vi "Begin.vi"(8 "error in":errorcluster) -> (0 "error out":errorcluster)   [LabVIEW 2017]
doc: "Called before other user functions, this VI is expected to open initial I/O refnums, load in file data, and do all program initialization. Notice that the <B>error out</B> terminal is simply used for data flow. Wiring it to other structures or subVIs ensures that this VI runs first."
uses:
  <vilib>/Rock Robotics/WPI/MotorControl/WPI_MotorControlDeviceRef.ctl
  <vilib>/Rock Robotics/WPI/MotorControl/WPI_MotorControlType.ctl
  <vilib>/Rock Robotics/SystemInterfaces/DIO/FPGA_DIOPWMChannel.ctl
  <vilib>/Rock Robotics/WPI/PWM/WPI_PWMDeadband.ctl
  <vilib>/Rock Robotics/SystemInterfaces/DIO/FPGA_DIOChannel.ctl
  <vilib>/Rock Robotics/WPI/DriverStation/WPI_DriverStationRobotMode2.ctl
  SwerveLibrary/Swerve Motors.ctl
  SwerveLibrary/Drive Motors.ctl
  SwerveLibrary/Controllers.ctl
  <vilib>/Rock Robotics/WPI/Joystick/WPI_JoystickDeviceEnum.ctl
  Arm Control/Arm Motor.ctl
  <vilib>/Rock Robotics/WPI/Solenoid/WPI_SolenoidChannel.ctl
  <vilib>/Rock Robotics/WPI/SafetyOutput/WPI_SafetyOutputConfigMenu.ctl
  Public/Documents/Cross The Road Electronics/Phoenix-LabVIEW/Motor Controller/Controls/CTRE_Phoenix_MotorControl_FeedbackDevice.ctl
  Pigeon IMU.ctl
  Robot Global Data.vi
  <vilib>/Rock Robotics/WPI/ThirdParty/Phoenix-LabVIEW/Pigeon IMU/CTRE_PigeonIMU_Open_CAN.vi
  Public/Documents/Cross The Road Electronics/Phoenix-LabVIEW/Pigeon IMU/CTRE_PigeonIMU_GetYPR.vi
  <vilib>/Rock Robotics/WPI/ThirdParty/Phoenix-LabVIEW/Motor Controller/Get/CTRE_Phoenix_MotorController_GetPulseWidthAll.vi
  <vilib>/Rock Robotics/WPI/Utilities/WPI_GetSetVariantRefNum.vi
  <vilib>/Rock Robotics/WPI/Solenoid/WPI_SolenoidOpenSingle.vi
  SwerveLibrary/Huskie Swerve.lvlib
panel:
  out "PhoenixMotorControlDevRef":T1={"DeviceStatus"={"status"=FALSE, "code"=0, "source"=""}, "Type"=enum."PWM", "PWM"={"PWM Channel"=enum."Invalid", "DeadBand"={"Name"="", "maxPositivePwm"=0, "minPositivePwm"=0, "centerPwm"=0, "maxNegativePwm"=0, "minNegativePwm"=0, "angularRange"=0}}, "CAN"={"Device Number"=0, "SetOutput VI Ref"=variant(refnum<vi> refnum), "GetOutput VI Ref"=variant(refnum<vi> refnum), "Enable VI Ref"=variant(refnum<vi> refnum), "Disable VI Ref"=variant(refnum<vi> refnum), "Data"=variant}, "Invert"=FALSE, "DIO PWM"={"PWM \"Enable\" Channel"=enum."Invalid", "DIOChannel"=enum."Invalid", "PWM Rate"=0.0}}
  out "Yaw Pitch Roll":cluster{"Yaw":dbl, "Pitch":dbl, "Roll":dbl}
  in  "PID gains":T6={"proportional gain (Kc)"=5.0, "integral time (Ti, min)"=0.0, "derivative time (Td, min)"=0.0} {"derivative time (Td, min)" format="%.3f"; "integral time (Ti, min)" format="%.8f"; "proportional gain (Kc)" format="%.8f"}
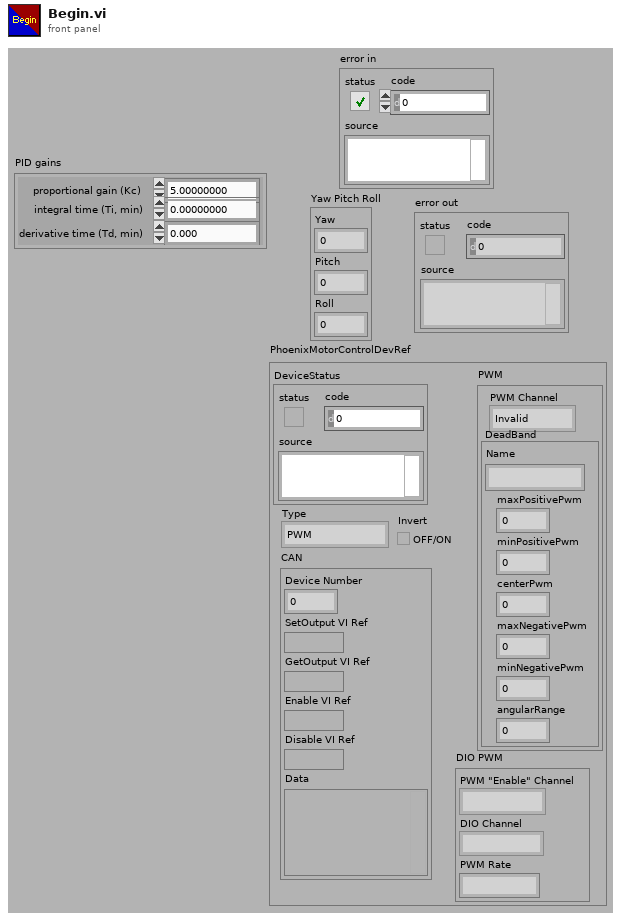
[diagram p1: front panel]
types:
  T1 = typedef "WPI_MotorControlDeviceRef.ctl" = cluster{"DeviceStatus":errorcluster, "Type":T2, "PWM":cluster{"PWM Channel":T3, "DeadBand":T4}, "CAN":cluster{"Device Number":u8, "SetOutput VI Ref":variant, "GetOutput VI Ref":variant, "Enable VI Ref":variant, "Disable VI Ref":variant, "Data":variant}, "Invert":bool, "DIO PWM":cluster{"PWM \"Enable\" Channel":T3, "DIOChannel":T5, "PWM Rate":dbl}}
  T2 = typedef "WPI_MotorControlType.ctl" = enum16{"PWM", "CAN", "DIO PWM"}
  T3 = typedef "FPGA_DIOPWMChannel.ctl" = enum8{"PWM 0", "PWM 1", "PWM 2", "PWM 3", "PWM 4", "PWM 5", "PWM 6", "PWM 7", "PWM 8", "PWM 9", "PWM MXP 0", "PWM MXP 1", "PWM MXP 2", "PWM MXP 3", "PWM MXP 4", "PWM MXP 5", "PWM MXP 6", "PWM MXP 7", "PWM MXP 8", "PWM MXP 9", "Invalid"}
  T4 = typedef "WPI_PWMDeadband.ctl" = cluster{"Name":string, "maxPositivePwm":i32, "minPositivePwm":i32, "centerPwm":i32, "maxNegativePwm":i32, "minNegativePwm":i32, "angularRange":u16}
  T5 = typedef "FPGA_DIOChannel.ctl" = enum8{"DIO 0", "DIO 1", "DIO 2", "DIO 3", "DIO 4", "DIO 5", "DIO 6", "DIO 7", "DIO 8", "DIO 9", "DIO MXP 0", "DIO MXP 1", "DIO MXP 2", "DIO MXP 3", "DIO MXP 4", "DIO MXP 5", "DIO MXP 6", "DIO MXP 7", "DIO MXP 8", "DIO MXP 9", "DIO MXP 10", "DIO MXP 11", "DIO MXP 12", "DIO MXP 13", "DIO MXP 14", "DIO MXP 15", "SPI Port CS1", "SPI Port CS2", "SPI Port CS3", "SPI Port MISO", "SPI Port MOSI", "Invalid"}
  T6 = cluster{"proportional gain (Kc)":dbl, "integral time (Ti, min)":dbl, "derivative time (Td, min)":dbl}
  T7 = typedef "WPI_SolenoidChannel.ctl" = enum8{"Solenoid 0", "Solenoid 1", "Solenoid 2", "Solenoid 3", "Solenoid 4", "Solenoid 5", "Solenoid 6", "Solenoid 7", "Invalid"}
  T8 = enum16{"Shoulder", "Forearm", "Grabber", "Extra"}[]
  T9 = typedef "Arm Motor.ctl" = enum16{"Shoulder Motor", "Forearm Motor"}
  T10 = typedef "WPI_JoystickDeviceEnum.ctl" = enum16{"USB 0", "USB 1", "USB 2", "USB 3", "USB 4", "USB 5"}
  T11 = typedef "Huskie Swerve.lvlib/Controllers.ctl" = enum16{"Joystick", "Buttons"}
  T12 = typedef "Huskie Swerve.lvlib/Drive Motors.ctl" = enum16{"Drive 1", "Drive 2", "Drive 3", "Drive 4"}
  T13 = typedef "Huskie Swerve.lvlib/Swerve Motors.ctl" = enum16{"Swerve 1", "Swerve 2", "Swerve 3", "Swerve 4"}
  T14 = typedef "WPI_DriverStationRobotMode2.ctl" = enum16{"Autonomous Disabled", "Autonomous Enabled", "Teleop Disabled", "Teleop Enabled", "Disconnected", "Finish", "Test Disabled", "Test Enabled", "Emergency Stopped"}
  T15 = typedef "WPI_SafetyOutputConfigMenu.ctl" = enum16{"Enable", "Disable"}
  T16 = typedef "CTRE_Phoenix_MotorControl_FeedbackDevice.ctl" = i8
  T17 = typedef "WPI_JoystickDevRef.ctl" = cluster{"Device":T10}
  T18 = typedef "Pigeon IMU.ctl" = enum16{"Pigeon IMU"}
  T19 = typedef "CTRE_PigeonIMU_DeviceRef.ctl" = cluster{"DeviceStatus":errorcluster, "Device Number":u8, "Type":T20, "Device ID":u32, "Handle":u64, "UsageFrame":u32, "Library Path":path}
  T20 = typedef "CTRE_PigeonIMU_ConnectionType.ctl" = u32
  T21 = typedef "WPI_CompressorDevRef.ctl" = cluster{"DevStatus":errorcluster, "Pneumatics Control Module":u8}
  T22 = typedef "WPI_SolenoidDevRef.ctl" = cluster{"DevStatus":errorcluster, "Pneumatics Control Module":u8, "Forward Solenoid Channel":T7, "Reverse Solenoid Channel":T7}
  T23 = typedef "WPI_DigitalInputDevRef.ctl" = cluster{"DevStatus":errorcluster, "DIO Channel":T5}
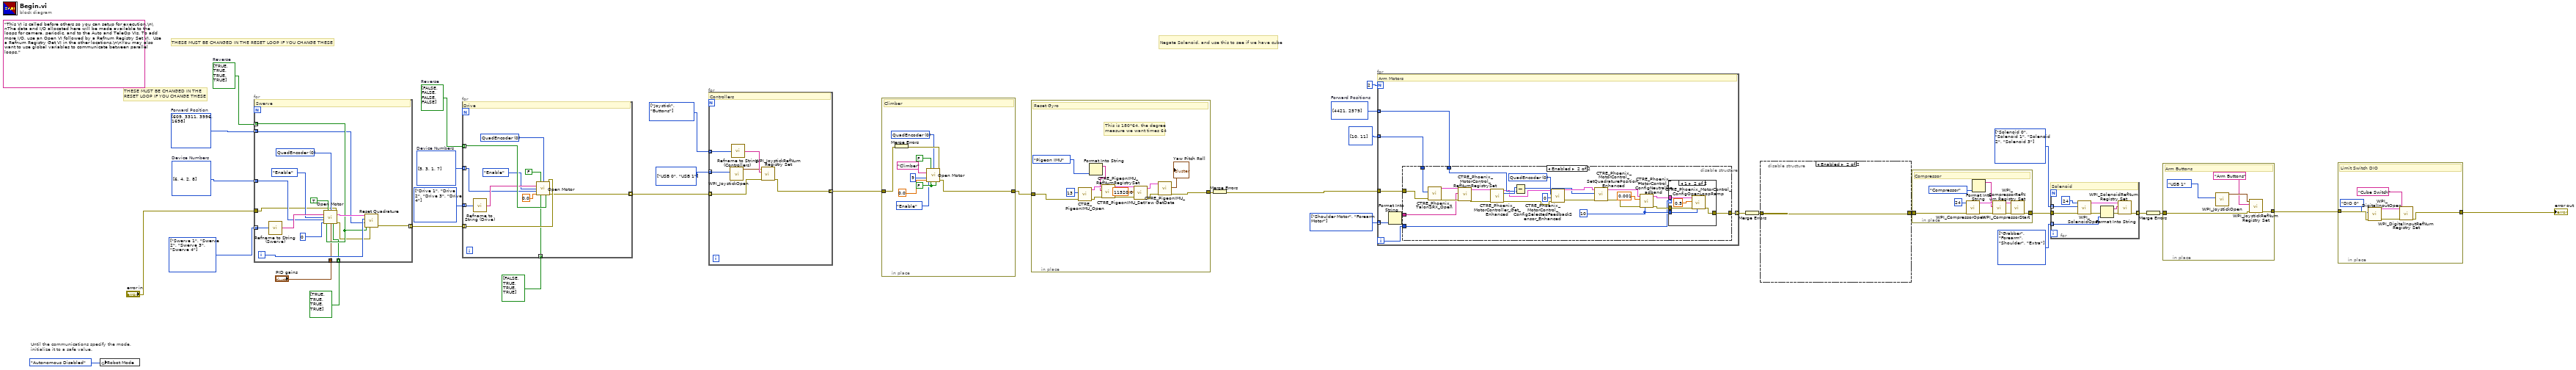
[diagram p0: block diagram]
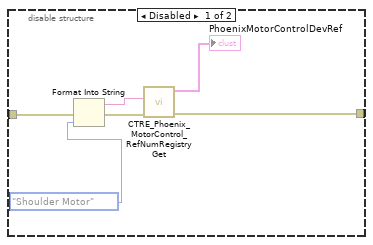
[diagram p2: hidden frame]
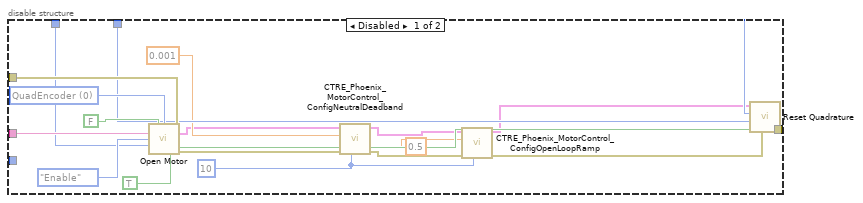
[diagram p3: hidden frame]
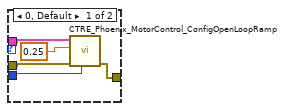
[diagram p4: hidden frame]
diagram:
  w8 = T7[] [enum."Solenoid 0", enum."Solenoid 1", enum."Solenoid 2", enum."Solenoid 3"] items=["Solenoid 0", "Solenoid 1", "Solenoid 2", "Solenoid 3", "Solenoid 4", "Solenoid 5", "Solenoid 6", "Solenoid 7", "Invalid"]
  w9 = T8 [enum."Grabber", enum."Forearm", enum."Shoulder", enum."Extra"] items=["Shoulder", "Forearm", "Grabber", "Extra"]
  w12 = T9[] [enum."Shoulder Motor", enum."Forearm Motor"] items=["Shoulder Motor", "Forearm Motor"]
  w15 = i32[] [4421, 2579]  # Forward Positions
  w22 = T10[] [enum."USB 0", enum."USB 1"] items=["USB 0", "USB 1", "USB 2", "USB 3", "USB 4", "USB 5"]
  w23 = T11[] [enum."Joystick", enum."Buttons"] items=["Joystick", "Buttons"]
  w25 = T12[] [enum."Drive 1", enum."Drive 2", enum."Drive 3", enum."Drive 4"] items=["Drive 1", "Drive 2", "Drive 3", "Drive 4"]
  w27 = i32[] [5, 3, 1, 7]  # Device Numbers
  w28 = bool[] [FALSE, FALSE, FALSE, FALSE]  # Reverse
  w29 = bool[] [TRUE, TRUE, TRUE, TRUE]  # Reverse
  w30 = T13[] [enum."Swerve 1", enum."Swerve 2", enum."Swerve 3", enum."Swerve 4"] items=["Swerve 1", "Swerve 2", "Swerve 3", "Swerve 4"]
  w31 = i32[] [6, 4, 2, 8]  # Device Numbers
  w33 = i32[] [609, 3311, 3996, 1698]  # Forward Position
  (unwired) "This VI is called before others so you can setup for execution.\n\nThe data and I/O allocated here will be made available to the loops for camera, periodic, and to the Auto and TeleOp VIs. To add more I/O, use an Open VI followed by a Refnum Registry Set VI.  Use a Refnum Registry Get VI in the other locations.\n\nYou may also want to use global variables to communicate between parallel loops."
  # "THESE MUST BE CHANGED IN THE \nRESET LOOP IF YOU CHANGE THESE"
  # "THESE MUST BE CHANGED IN THE RESET LOOP IF YOU CHANGE THESE"
  # "Negate Solenoid, and use this to see if we have cube"
  # "Until the communications specify the mode,\ninitialize it to a safe value."
  n1 = global write "Robot Global Data.vi" "Robot Mode"(WPI_DriverStationRobotMode2."Autonomous Disabled" ("Robot Mode")) -> ()
  n2 = for {
    tunnel: w33 -> [w39] mode=indexing
    tunnel: "error in" -> [w43]
    tunnel: w31 -> [w48] mode=indexing
    tunnel: w30 -> [w50] mode=indexing
    tunnel: w29 -> [w40] mode=indexing
    tunnel: [w37] -> w26 mode=indexing
    tunnel: "PID gains" -> [w36]
    tunnel: bool[] [TRUE, TRUE, TRUE, TRUE] -> [w35] mode=indexing
    i -> [w41]
    w44 = T16 0 items=["None"=-1, "QuadEncoder"=0, "Analog"=2, "Tachometer"=4, "Pulse Width Encoded Position"=8, "Sensor Sum (S0 + S1)"=9, "Sensor Difference (D0 - D1)"=10, "Remote Source 0"=11, "Remote Source 1"=12, "Software Emulated"=15] ("Feedback Reference")
    # "Swerve"
    n3 = call "Refname to String (Swerve).vi"("Enum"=w50) -> ("String"=w49:string)
    n4 = call "Open Motor.vi"("PID?"=TRUE, "Feedback Reference"=w44, "error in"=w43, "refnum name"=w49, "mode (safety config)"=WPI_SafetyOutputConfigMenu."Enable", "CAN Device Number"=w48, "Set sensor position"=0, "Reverse Feedback Sensor"=w40, "PID gains"=w36, "Invert Power"=w35) -> ("CAN Talon SRX Ref"=w42:T1, "error out"=w38:errorcluster)  [unwired: 4 in]
    n5 = call "Reset Quadrature.vi"("error in"=w38, "Reverse?"=w40, "Forward Position"=w39, "Module Number"=w41, "CAN Talon SRX Ref"=w42) -> ("error out"=w37:errorcluster)  [unwired: 5 in, 1 out]
  }
  n6 = for {
    tunnel: [w52] -> w24 mode=indexing
    tunnel: w28 -> [w60] mode=indexing
    tunnel: w27 -> [w58] mode=indexing
    tunnel: w26 -> [w53] mode=indexing
    tunnel: w25 -> [w61] mode=indexing
    tunnel: bool[] [FALSE, TRUE, TRUE, TRUE] ("Reverse Feedback Sensor") -> [w51] mode=indexing
    w54 = T16 0 items=["None"=-1, "QuadEncoder"=0, "Analog"=2, "Tachometer"=4, "Pulse Width Encoded Position"=8, "Sensor Sum (S0 + S1)"=9, "Sensor Difference (D0 - D1)"=10, "Remote Source 0"=11, "Remote Source 1"=12, "Software Emulated"=15] ("Feedback Reference")
    # "Drive"
    n7 = call "Refname to String (Drive).vi"("Enum"=w61) -> ("resulting string"=w59:string)
    n8 = call "Open Motor.vi"("PID?"=FALSE, "Feedback Reference"=w54, "error in"=w53, "refnum name"=w59, "mode (safety config)"=WPI_SafetyOutputConfigMenu."Enable", "CAN Device Number"=w58, "Set sensor position"=0.0, "Reverse Feedback Sensor"=w51, "Invert Power"=w60) -> ("error out"=w52:errorcluster)  [unwired: 5 in, 1 out]
  }
  n9 = for {
    tunnel: [w62] -> w18 mode=indexing
    tunnel: w24 -> [w63] mode=indexing
    tunnel: w23 -> [w66] mode=indexing
    tunnel: w22 -> [w67] mode=indexing
    # "Controllers"
    n10 = call <vilib>:"WPI_JoystickOpen.vi"("JoystickDevice"=w67) -> ("JoystickDevRef"=w64:T17)  [unwired: 10 in]
    n11 = call "Refname to String (Controllers).vi"("Enum"=w66) -> ("resulting string"=w65:string)
    n12 = call <vilib>:"WPI_JoystickRefNum Registry Set.vi"("error in (no error)"=w63, "refnum name"=w65, "JoystickDevRef"=w64) -> ("error out"=w62:errorcluster)  [unwired: 7 in, 1 out]
  }
  n13 = in-place "In Place Element Structure" {
    in-place-border: w18 -> [w76]
    in-place-border: [w68] -> w17
    w72 = T16 0 items=["None"=-1, "QuadEncoder"=0, "Analog"=2, "Tachometer"=4, "Pulse Width Encoded Position"=8, "Sensor Sum (S0 + S1)"=9, "Sensor Difference (D0 - D1)"=10, "Remote Source 0"=11, "Remote Source 1"=12, "Software Emulated"=15] ("Feedback Reference")
    w73 = FALSE ("Reverse Feedback Sensor")
    # "Climber"
    n14 = Merge Errors(w76) -> (w75:errorcluster)
    n15 = call "Open Motor.vi"("PID?"=FALSE, "Feedback Reference"=w72, "error in"=w75, "refnum name"="Climber", "mode (safety config)"=WPI_SafetyOutputConfigMenu."Enable", "CAN Device Number"=u8 9, "Set sensor position"=0.0, "Reverse Feedback Sensor"=w73, "Invert Power"=w73) -> ("error out"=w68:errorcluster)  [unwired: 5 in, 1 out]
  }
  n16 = in-place {
    in-place-border: w17 -> [w89]
    in-place-border: [w79] -> w16
    # "This is 180*64, the degree\nmeasure we want times 64"
    # "Reset Gyro"
    n17 = call-poly <vilib>:"CTRE_PigeonIMU_Open.vi"("error in"=w89, "Device Number"=u8 13) -> ("error out"=w87:errorcluster, "PigeonIMUDevRef"=w86:T19)  [unwired: 8 in]
    n18 = Format Into String(Pigeon_IMU."Pigeon IMU") -> (resulting string=w85:string)  [unwired: 3 in, 1 out]
    n19 = call <vilib>:"CTRE_PigeonIMU_RefNumRegistrySet.vi"("error in (no error)"=w87, "refnum name"=w85, "PigeonIMUDevRef"=w86) -> ("error out"=w84:errorcluster, "PigeonIMUDevRef"=w83:T19)  [unwired: 7 in]
    n20 = call <vilib>:"CTRE_PigeonIMU_SetYaw.vi"("error in (no error)"=w84, "Value"=11520.0, "PigeonIMUDevRef"=w83) -> ("error out"=w80:errorcluster, "PigeonIMUDevRef"=w81:T19)  [unwired: 7 in]
    n21 = call-poly "CTRE_PigeonIMU_GetData.vi"("error in (no error)"=w80, "PigeonIMUDevRef"=w81) -> ("error out"=w79:errorcluster, "Yaw Pitch Roll"=→"Yaw Pitch Roll":cluster{"Yaw":dbl, "Pitch":dbl, "Roll":dbl})  [unwired: 7 in, 1 out]
  }
  n22 = Merge Errors(w16) -> (w3:errorcluster)
  n23 = for {
    N: 2 -> [_]
    tunnel: w3 -> [w97]
    tunnel: w15 -> [w94] mode=indexing
    tunnel: i32[] [10, 11] -> [w93] mode=indexing
    tunnel: w12 -> [w95] mode=indexing
    tunnel: [w92] -> w7 mode=indexing
    i -> [w91]
    # "Arm Motors"
    n24 = Format Into String(w95) -> (resulting string=w96:string)  [unwired: 3 in, 1 out]
    n25 = disable-structure shown="Enabled" {
      disable-tunnel: w97 -> [w116 w139]
      disable-tunnel: w96 -> [w113 w136]
      disable-tunnel: w94 -> [w109 w130]
      disable-tunnel: w93 -> [w108 w140]
      disable-tunnel: [w104 w119] -> w92
      disable-tunnel: w91 -> [_ w117]
      frame Disabled {
        w100 = u32 10 ("timeoutMs")
        w114 = T16 0 items=["None"=-1, "QuadEncoder"=0, "Analog"=2, "Tachometer"=4, "Pulse Width Encoded Position"=8, "Sensor Sum (S0 + S1)"=9, "Sensor Difference (D0 - D1)"=10, "Remote Source 0"=11, "Remote Source 1"=12, "Software Emulated"=15] ("Feedback Reference")
        n26 = call "Open Motor.vi"("PID?"=FALSE, "Feedback Reference"=w114, "error in"=w116, "refnum name"=w113, "mode (safety config)"=WPI_SafetyOutputConfigMenu."Enable", "CAN Device Number"=w108, "Invert Power"=TRUE) -> ("CAN Talon SRX Ref"=w106:T1, "Reverse Feedback Sensor"=w110:bool, "error out"=w105:errorcluster)  [unwired: 6 in]
        n27 = call <vilib>:"CTRE_Phoenix_MotorControl_ConfigNeutralDeadband.vi"("timeoutMs"=w100, "error in (no error)"=w105, "Percent Deadband"=0.001, "PhoenixMotorControlDevRef"=w106) -> ("error out"=w103:errorcluster, "PhoenixMotorControlDevRef"=w101:T1)  [unwired: 6 in]
        n28 = call <vilib>:"CTRE_Phoenix_MotorControl_ConfigOpenLoopRamp.vi"("timeoutMs"=w100, "error in (no error)"=w103, "secondsFromNeutralToFull"=0.5, "PhoenixMotorControlDevRef"=w101) -> ("error out"=w102:errorcluster, "PhoenixMotorControlDevRef"=w98:T1)  [unwired: 6 in]
        n29 = call "Reset Quadrature.vi"("error in"=w102, "Reverse?"=w110, "Forward Position"=w109, "Module Number"=w108, "CAN Talon SRX Ref"=w98) -> ("error out"=w104:errorcluster)  [unwired: 5 in, 1 out]
      }
      frame Enabled {
        w123 = u32 10 ("timeoutMs")
        w135 = T16 0 items=["None"=-1, "QuadEncoder"=0, "Analog"=2, "Tachometer"=4, "Pulse Width Encoded Position"=8, "Sensor Sum (S0 + S1)"=9, "Sensor Difference (D0 - D1)"=10, "Remote Source 0"=11, "Remote Source 1"=12, "Software Emulated"=15] ("Feedback Device")
        n30 = call "CTRE_Phoenix_TalonSRX_Open.vi"("error in"=w139, "Device Number"=w140) -> ("error out"=w138:errorcluster, "CAN Talon SRX Ref"=w137:T1)  [unwired: 8 in]
        n31 = call <vilib>:"CTRE_Phoenix_MotorControl_RefNumRegistrySet.vi"("error in (no error)"=w138, "refnum name"=w136, "PhoenixMotorControlDevRef"=w137) -> ("error out"=w126:errorcluster, "PhoenixMotorControlDevRef"=w125:T1)  [unwired: 7 in]
        n32 = call-poly <vilib>:"CTRE_Phoenix_MotorController_Get_Enhanced.vi"("PhoenixMotorControlDevRef"=w125, "error in"=w126) -> ("PhoenixMotorControlDevRef"=w129:T1, "Pulse Width Position"=w131:i32, "error out"=w127:errorcluster)  [unwired: 8 in, 3 out]
        n33 = Subtract(x=w131, y=w130) -> (x-y=w128:i32)
        n34 = call "CTRE_Phoenix_MotorControl_ConfigSelectedFeedbackSensor_Enhanced.vi"("error in (no error)"=w127, "pidLoopIdx"=0, "Feedback Device"=w135, "PhoenixMotorControlDevRef"=w129) -> ("error out"=w132:errorcluster, "PhoenixMotorControlDevRef"=w133:T1)  [unwired: 6 in]
        n35 = call <vilib>:"CTRE_Phoenix_MotorControl_SetQuadraturePosition_Enhanced.vi"("error in (no error)"=w132, "New Position"=w128, "PhoenixMotorControlDevRef"=w133) -> ("error out"=w122:errorcluster, "PhoenixMotorControlDevRef"=w121:T1)  [unwired: 7 in]
        n36 = call <vilib>:"CTRE_Phoenix_MotorControl_ConfigNeutralDeadband.vi"("timeoutMs"=w123, "error in (no error)"=w122, "Percent Deadband"=0.001, "PhoenixMotorControlDevRef"=w121) -> ("error out"=w124:errorcluster, "PhoenixMotorControlDevRef"=w120:T1)  [unwired: 6 in]
        n37 = case shown="1" w117 {
          tunnel: w124 -> [w142 w150]
          tunnel: w123 -> [w143 w149]
          tunnel: w120 -> [w141 w147]
          tunnel: [w144 w146] -> w119
          frame 0, Default {
            n38 = call <vilib>:"CTRE_Phoenix_MotorControl_ConfigOpenLoopRamp.vi"("timeoutMs"=w143, "error in (no error)"=w142, "secondsFromNeutralToFull"=0.25, "PhoenixMotorControlDevRef"=w141) -> ("error out"=w144:errorcluster)  [unwired: 6 in, 1 out]
          }
          frame 1 {
            n39 = call <vilib>:"CTRE_Phoenix_MotorControl_ConfigOpenLoopRamp.vi"("timeoutMs"=w149, "error in (no error)"=w150, "secondsFromNeutralToFull"=0.5, "PhoenixMotorControlDevRef"=w147) -> ("error out"=w146:errorcluster)  [unwired: 6 in, 1 out]
          }
        }
      }
    }
  }
  n40 = Merge Errors(w7) -> (w5:errorcluster)
  n41 = disable-structure shown="Enabled" {
    disable-tunnel: w5 -> [w156 w157]
    disable-tunnel: [w154 w157] -> w4
    frame Disabled {
      n42 = Format Into String(error in=w156, Arm_Motor."Shoulder Motor" ("Enum")) -> (resulting string=w152:string, error out=w155:errorcluster)  [unwired: 2 in]
      n43 = call "CTRE_Phoenix_MotorControl_RefNumRegistryGet.vi"("error in (no error)"=w155, "refnum name"=w152) -> ("error out"=w154:errorcluster, "PhoenixMotorControlDevRef"=→"PhoenixMotorControlDevRef":T1)  [unwired: 8 in]
    }
    frame Enabled {
    }
  }
  n44 = in-place "In Place Element Structure" {
    in-place-border: w4 -> [w165]
    in-place-border: [w158] -> w11
    # "Compressor"
    n45 = call <vilib>:"WPI_CompressorOpen.vi"("Pneumatics Control Module (0)"=u8 24, "error in (no error)"=w165) -> ("CompressorDevRef"=w164:T21, "error out"=w161:errorcluster)  [unwired: 12 in]
    n46 = Format Into String(enum16{"Compressor"}."Compressor" ("Enum")) -> (resulting string=w162:string)  [unwired: 3 in, 1 out]
    n47 = call <vilib>:"WPI_CompressorRefNum Registry Set.vi"("error in (no error)"=w161, "refnum name"=w162, "CompressorDevRef"=w164) -> ("error out"=w160:errorcluster, "CompressorDevRef"=w159:T21)  [unwired: 7 in]
    n48 = call <vilib>:"WPI_CompressorStart.vi"("error in (no error)"=w160, "CompressorDevRef"=w159) -> ("error out"=w158:errorcluster)  [unwired: 8 in, 1 out]
  }
  n49 = for {
    tunnel: w11 -> [w175]
    tunnel: [w170] -> w10 mode=indexing
    tunnel: w9 -> [w169] mode=indexing
    tunnel: w8 -> [w167] mode=indexing
    # "Solenoid"
    n50 = call-poly <vilib>:"WPI_SolenoidOpen.vi"("error in (no error)"=w175, "Solenoid Channel"=w167, "Pneumatics Control Module (0)"=u8 24) -> ("error out"=w173:errorcluster, "SolenoidDevRef"=w172:T22)  [unwired: 7 in]
    n51 = Format Into String(error in=w173, w169) -> (resulting string=w171:string, error out=w174:errorcluster)  [unwired: 2 in]
    n52 = call <vilib>:"WPI_SolenoidRefNum Registry Set.vi"("error in (no error)"=w174, "refnum name"=w171, "SolenoidDevRef"=w172) -> ("error out"=w170:errorcluster)  [unwired: 7 in, 1 out]
  }
  n53 = Merge Errors(w10) -> (w6:errorcluster)
  n54 = in-place "In Place Element Structure" {
    in-place-border: w6 -> [w177]
    in-place-border: [w176] -> w2
    # "Arm Buttons"
    n55 = call <vilib>:"WPI_JoystickOpen.vi"("JoystickDevice"=WPI_JoystickDeviceEnum."USB 1") -> ("JoystickDevRef"=w179:T17)  [unwired: 10 in]
    n56 = call <vilib>:"WPI_JoystickRefNum Registry Set.vi"("error in (no error)"=w177, "refnum name"="Arm Buttons", "JoystickDevRef"=w179) -> ("error out"=w176:errorcluster)  [unwired: 7 in, 1 out]
  }
  n57 = in-place "In Place Element Structure" {
    in-place-border: w2 -> [w185]
    in-place-border: [w184] -> w1
    # "Limit Switch DIO"
    n58 = call <vilib>:"WPI_DigitalInputOpen.vi"("error in (no error)"=w185, "DIO Channel"=FPGA_DIOChannel."DIO 0") -> ("error out"=w186:errorcluster, "DigitalInputDevRef"=w183:T23)  [unwired: 8 in]
    n59 = call <vilib>:"WPI_DigitalInputRefNum Registry Set.vi"("error in (no error)"=w186, "refnum name"="Cube Switch", "DigitalInputDevRef"=w183) -> ("error out"=w184:errorcluster)  [unwired: 7 in, 1 out]
  }
  "error out" <- w1
